vi "OpenInterface.vi"(8 "error in (no error)":errorcluster, 9 "handle":i64) -> (0 "error out":errorcluster, 2 "return type":i32)   [LabVIEW 2013, in "MvCameraControl.lvlib"]
uses:
  MvCameraControl.lvlib
  MvCameraControl.dll
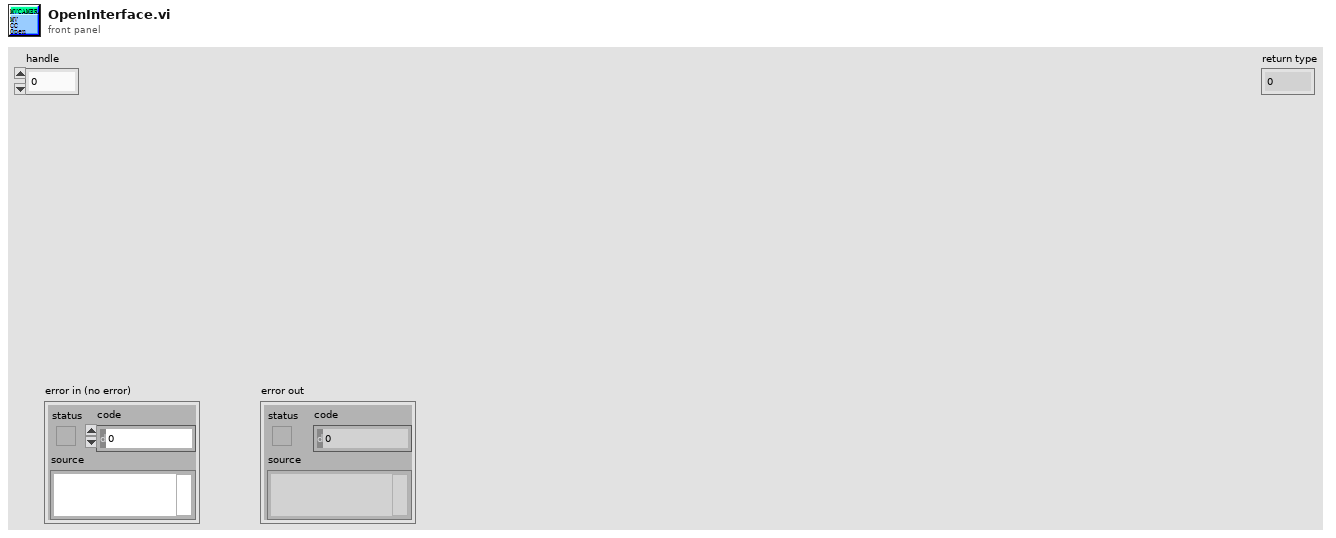
[diagram p1: front panel]
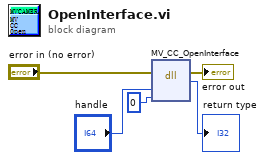
[diagram p0: block diagram]
diagram:
  n1 = dll-call lib="MvCameraControl.*" fn="MV_CC_OpenInterface"(error in="error in (no error)", "handle"="handle", "reserved"=i8 0) -> (error out=→"error out":errorcluster, "return type"=→"return type":i32)  [unwired: 4 in, 1 out]
